vi "USRP Copy Reference for Preview.vi"(8 "error in (no error)":errorcluster, 10 "FPGA FIFO Reference in":refnum<data-value>, 11 "Data Preview Reference in":refnum<data-value>) -> (0 "error out":errorcluster, 2 "FPGA FIFO Reference out":refnum<data-value>, 3 "Data Preview Reference out":refnum<data-value>)   [LabVIEW 2016]
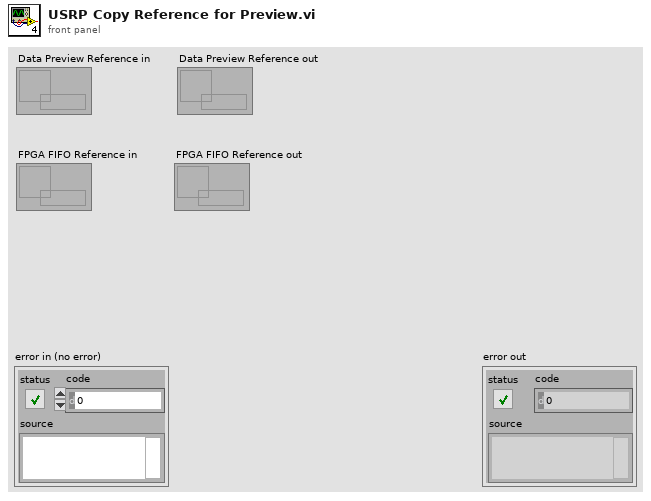
[diagram p1: front panel]
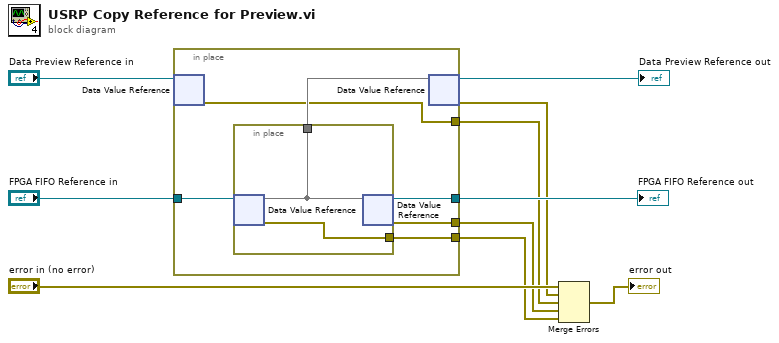
[diagram p0: block diagram]
diagram:
  n1 = in-place {
    in-place-border: [w14] -> w3
    in-place-border: [w12] -> w2
    in-place-border: "FPGA FIFO Reference in" -> [w16]
    in-place-border: [w13] -> w1
    in-place-border: [w11] -> w5
    n2 = in-place-dvr #1("Data Preview Reference in") -> (w14:errorcluster)  [unwired: 1 out]
    n3 = in-place {
      in-place-border: [w18] -> w15
      in-place-border: [w17] -> w13
      n4 = in-place-dvr #2(w16) -> (w18:u64[], w17:errorcluster)
      n5 = in-place-dvr #2(w18) -> (w11:refnum<data-value>, w12:errorcluster)
    }
    n6 = in-place-dvr #1(w15) -> (→"Data Preview Reference out":refnum<data-value>, w4:errorcluster)
  }
  "FPGA FIFO Reference out" <- w5
  n7 = Merge Errors("error in (no error)", w4, w3, w2, w1) -> (→"error out":errorcluster)
